vi "Join Strings.vi"(6 "Separator (,)":string=",", 10 "Strings In":string[](array[string])) -> (2 "String":string)   [LabVIEW 2020, in "String Manipulation.lvlib"]
uses:
  <vilib>/gpm_packages/@cs/linked-list/Source/String Manipulation/String Manipulation.lvlib
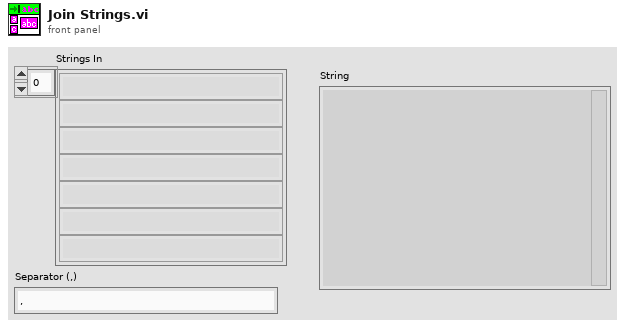
[diagram p1: front panel]
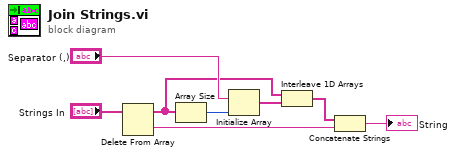
[diagram p0: block diagram]
diagram:
  n1 = Delete From Array(array="Strings In") -> (deleted portion=w2:string, array with subset deleted=w5:string[])  [unwired: 2 in]
  n2 = Array Size(array=w5) -> (size(s)=w6:i32)
  n3 = Initialize Array("Separator (,)", w6) -> (w4:string[])
  n4 = Interleave 1D Arrays(w5, w4) -> (w3:string[])
  n5 = Concatenate Strings(w3, w2) -> (→"String":string)
